vi "MotorBlockPI_FPGA.vi"(1 "Encoder":T1(ring), 3 "STOP":bool, 5 "Value":dbl, 7 "Custom FPGA Reference In":refnum<k20>, 9 "Speed":dbl, 11 "error in (no error)":errorcluster, 12 "Type":enum16{"Iterations", "Counts", "Time"}(ring), 13 "Motor":T2(ring), 14 "Sentido":bool) -> (4 "Waveform \nChart":dbl[][](graph), 10 "FPGA VI Reference Out":refnum<k20>, 15 "error out":errorcluster)   [LabVIEW 2017]
doc: "This program is an PI counts based program usgin only the FPGA customized encoders. \nIt works using counts, degrees, iterations, time or rotations.\nEach iteration delates 5 ms. You must to use with VI without a while loop."
uses:
  <vilib>/Platform/TimedLoop/XDataNode/timing_clust.ctl
  <vilib>/Platform/TimedLoop/XDataNode/nitl_modes.ctl
  <vilib>/Platform/TimedLoop/XDataNode/wakeup.ctl
  <vilib>/Utility/error.llb/Error Cluster From Error Code.vi
  <vilib>/rvi/errors/niLvFpgaAdjustHostInterfaceError.vi
  <vilib>/myRIO/Common/Instrument Driver Framework/myRIO v1.0/DIO/vis/myRIO v1.0 Write DIO.vi
  <vilib>/myRIO/Common/Instrument Driver Framework/myRIO v1.0/PWM/vis/myRIO v1.0 Write PWM.vi
  <vilib>/Platform/TimedLoop/XDataNode/XDataNode.xnode
  <vilib>/rvi/interface/nirviReadWriteControl/nirviReadWriteControl.xnode
  <vilib>/myRIO/Instrument Drivers/Onboard IO/PWM/PWM.lvlib
  <vilib>/myRIO/Instrument Drivers/Onboard IO/DIO/DIO.lvlib
  <vilib>/Platform/TimedLoop/XDataNode/XDNodeRunTimeDep.lvlib
  NiFpgaLv.dll
  <vilib>/rvi/interface/Simulation/niFpgaSimulationCallBeginRW.vi
panel:
  # "Este programa implementa un control por odometría usando únicamente los \nencoders de la FPGA. \nWRO 2018 @ Tecnológico de Costa Rica"
  # "El programa puede hacer funcionar los motores por tiempo, \niteraciones, grados, rotaciones o cuentas puras. \nParametros de entrada:\nType: Selecciona el modo desea para operar el programa:\n        \n            2. Time:     Detiene el motor depués de transcurrido el \n                                tiempo deseado.\n            3. Iteration:     Detiene el motor depués de transcurrido una\n                                cantidad de iteraciones.\n             5. Counts:  Detiene el motor depués de alcanzada la posición \n                                 en cuentas deseada.\nValue: Indica el valor de la condición de parada deseada.\nMotor: Selecciona el puerto y el motor.\nSentido: Selecciona el sentido de giro.\nFPGA Reference In: Selecciona la referencia al programa de FPGA.\nFPGA Reference Out: Envía la referencia al programa de FPGA.\nError I/O: Maneja las entadas y salidas de error.\nEncoder: Selecciona la entrada a utilizar como encoder. Los números \nrepresentan el número de DIO que se deben conectar, y siempre el número \nmás pequeño representa la fase A."
  # "Horario"
  # "Antihorario"
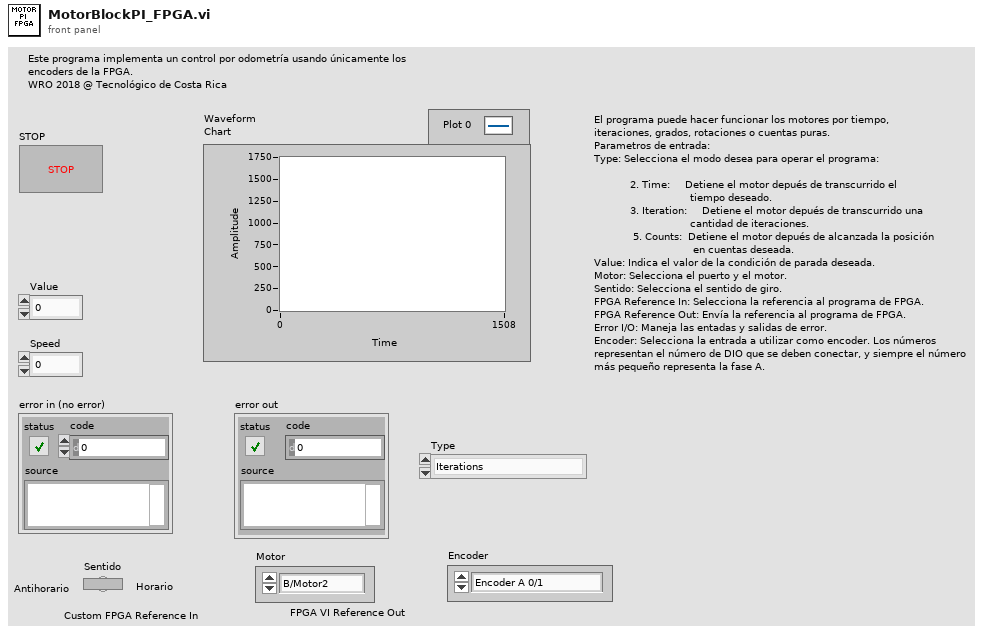
[diagram p1: front panel]
types:
  T1 = enum16{"Encoder A 0/1", "Encoder A 11/12", "Encoder A 4/13", "Encoder B 0/1", "Encoder B 11/12", "Encoder B 4/13", "Encoder C 4/6", "Encoder C 0/2"}
  T2 = enum16{"B/Motor2", "B/Motor1", "A/Motor2", "A/Motor1"}
  T3 = typedef "XDNodeRunTimeDep.lvlib/timing_clust.ctl" = cluster{"Expected End [f-1]":u64, "Actual End [f-1]":u64, "Finished Late? [f-1]":bool, "Expected End [i-1]":u64, "Actual End [i-1]":u64, "Finished Late? [i-1]":bool, "Expected Start [i]":u64, "Actual Start [i]":u64, "Expected Start [f]":u64, "Actual Start [f]":u64, "Source Name":string, "Structure Name":string, "Period":i64, "Deadline":i64, "Offset":i64, "Start":i64, "Priority":i32, "Timeout":i32, "Mode":T4, "Wakeup Reason":T5, "Error":errorcluster, "Source Type":string, "Secondary Source Type":string, "Global End Time":u64, "Global Start Time":u64, "Frame Duration":u64, "Iteration Duration":u64, "Assigned CPU":i32, "I/O Scan Engine Mode":u32}
  T4 = typedef "XDNodeRunTimeDep.lvlib/nitl_modes.ctl" = enum32{"No Change", "Process missed periods, maintain original phase", "Discard missed periods, maintain original phase", "Process missed periods, ignore original phase", "Discard missed periods, ignore original phase"}
  T5 = typedef "XDNodeRunTimeDep.lvlib/wakeup.ctl" = enum32{"Normal", "Aborted", "Asynchronous wakeup", "Timing source error", "Timed loop error", "Timeout"}
  T6 = typedef "DIO.lvlib/DIO Reference.ctl" = cluster{"myRIO Reference":T7, "DIO Channels List":T11}
  T7 = typedef "myRIO Generic Hardware Reference.ctl" = cluster{"myRIO Model":T8, "myRIO Hardware Reference":T9}
  T8 = typedef "Hardware Version Enum.ctl" = enum16{"Unknown", "myRIO-1900", "myRIO-1950", "roboRIO", "NI ELVIS RIO CM"}
  T9 = typedef "myRIO v1.0 Reference.ctl" = cluster{"Generic FPGA Reference":T10, "Allow multiple opens":bool}
  T10 = typedef "Generic FPGA Reference.ctl" = refnum<k20>
  T11 = typedef "DIO Channels List.ctl" = T12[]
  T12 = typedef "DIO Channels Enum.ctl" = enum16{"Not Connected", "C/DIO0", "C/DIO1", "C/DIO2", "C/DIO3", "C/DIO4", "C/DIO5", "C/DIO6", "C/DIO7", "A/DIO0", "A/DIO1", "A/DIO2", "A/DIO3", "A/DIO4", "A/DIO5", "A/DIO6", "A/DIO7", "A/DIO8", "A/DIO9", "A/DIO10", "A/DIO11", "A/DIO12", "A/DIO13", "A/DIO14", "A/DIO15", "B/DIO0", "B/DIO1", "B/DIO2", "B/DIO3", "B/DIO4", "B/DIO5", "B/DIO6", "B/DIO7", "B/DIO8", "B/DIO9", "B/DIO10", "B/DIO11", "B/DIO12", "B/DIO13", "B/DIO14", "B/DIO15", "LED0", "LED1", "LED2", "LED3", "Button0", "DIO/DIO0", "DIO/DIO1", "DIO/DIO2", "DIO/DIO3", "DIO/DIO4", "DIO/DIO5", "DIO/DIO6", "DIO/DIO7", "DIO/DIO8", "DIO/DIO9", "SPI/CS0", "SPI/CS1", "SPI/CS2", "SPI/CS3", "LED RADIO (Green)", "LED RADIO (Red)", "LED COMM (Green)", "LED COMM (Red)", "LED MODE (Green)", "LED MODE (Red)"}
  T13 = typedef "PWM.lvlib/PWM Reference.ctl" = cluster{"myRIO Reference":T7, "PWM Channels Enum":T14, "PWM Configuration":T15}
  T14 = typedef "PWM Channels Enum.ctl" = enum16{"Not Connected", "C/PWM0", "C/PWM1", "A/PWM0", "A/PWM1", "A/PWM2", "B/PWM0", "B/PWM1", "B/PWM2", "PWM/PWM0", "PWM/PWM1", "PWM/PWM2", "PWM/PWM3", "PWM/PWM4", "PWM/PWM5", "PWM/PWM6", "PWM/PWM7", "PWM/PWM8", "PWM/PWM9"}
  T15 = typedef "PWM.lvlib/PWM Configuration.ctl" = cluster{"Frequency":dbl, "Duty Cycle":dbl}
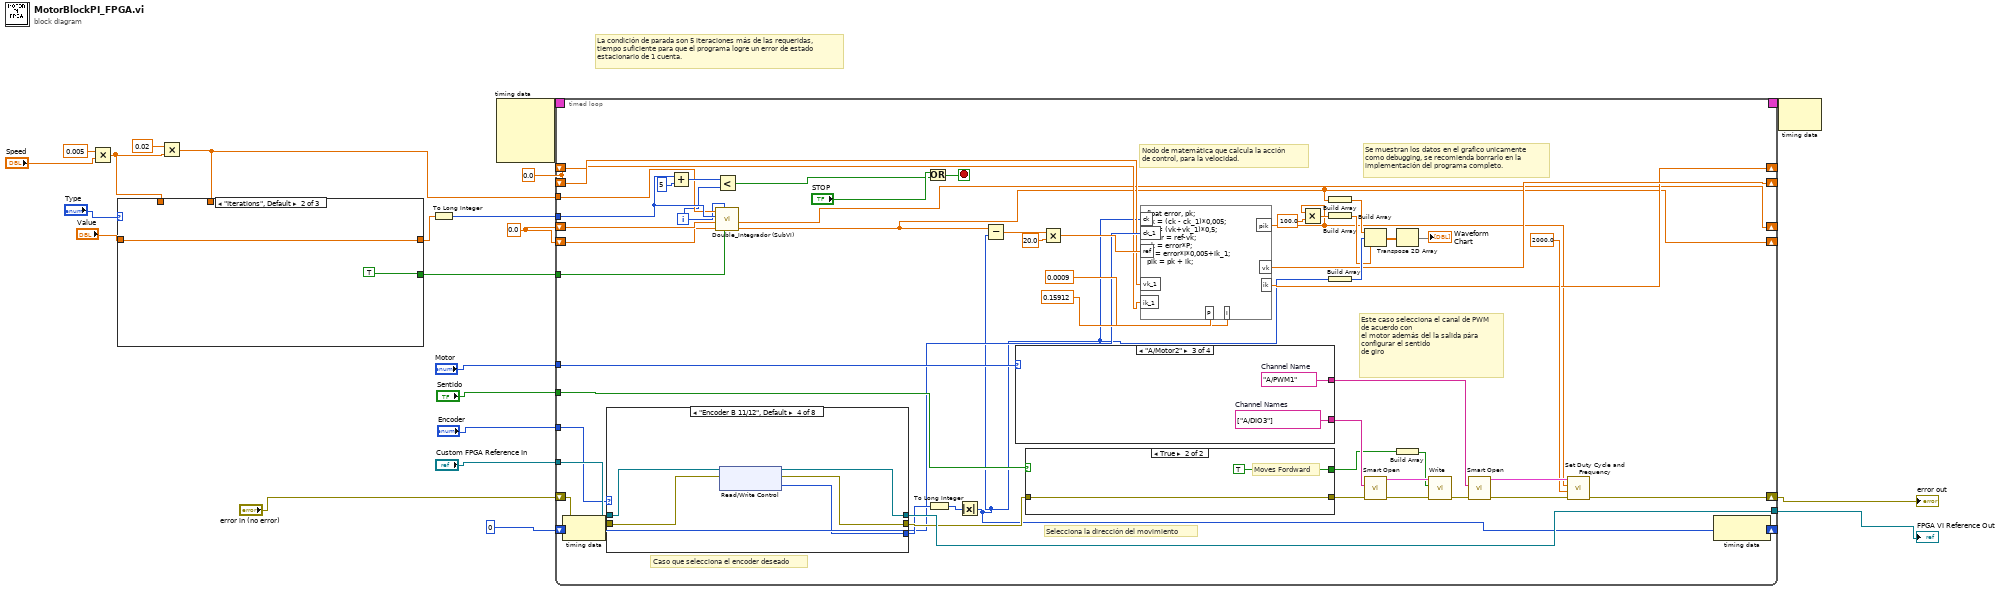
[diagram p0: block diagram]
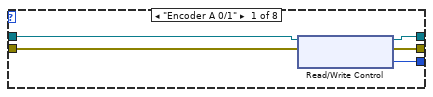
[diagram p2: hidden frame]
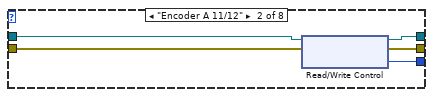
[diagram p3: hidden frame]
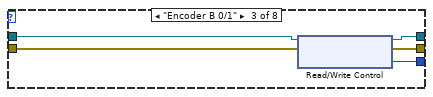
[diagram p4: hidden frame]
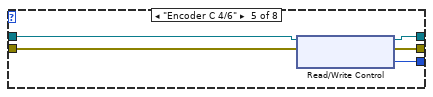
[diagram p5: hidden frame]
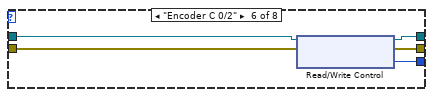
[diagram p6: hidden frame]
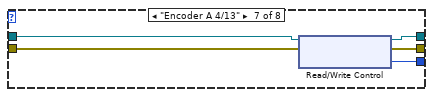
[diagram p7: hidden frame]
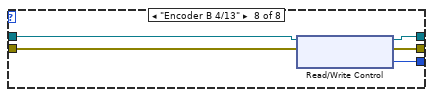
[diagram p8: hidden frame]
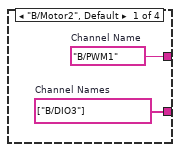
[diagram p9: hidden frame]
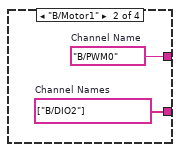
[diagram p10: hidden frame]
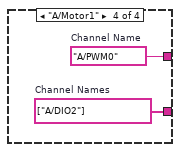
[diagram p11: hidden frame]
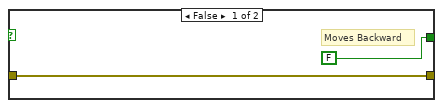
[diagram p12: hidden frame]
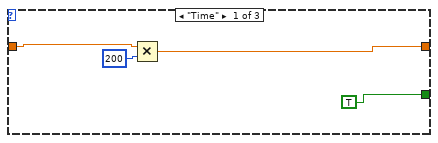
[diagram p13: hidden frame]
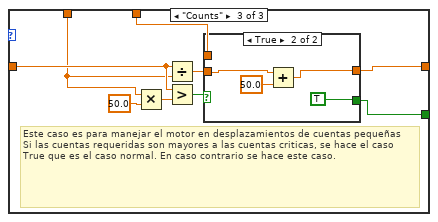
[diagram p14: hidden frame]
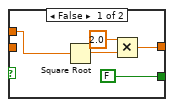
[diagram p15: hidden frame]
diagram:
  w17 = 0.0
  w11 = 0.0
  # "La condición de parada son 5 iteraciones más de las requeridas,\ntiempo suficiente para que el programa logre un error de estado\nestacionario de 1 cuenta."
  n1 = Multiply(x=0.005, y="Speed") -> (x*y=w4:dbl)
  n2 = Multiply(x=0.02, y=w4) -> (x*y=w2:dbl)
  n3 = case shown="\"Iterations\", Default" "Type" {
    tunnel: "Value" -> [w24 w27 w32]
    tunnel: w4 -> [_ _ w30]
    tunnel: [w25 w27 w35] -> w10
    tunnel: [TRUE TRUE w33] -> w8
    tunnel: w2 -> [_ _ w29]
    frame "Time" {
      n4 = Multiply(x=w24, y=200) -> (x*y=w25:dbl)
    }
    frame "Iterations", Default {
    }
    frame "Counts" {
      # "Este caso es para manejar el motor en desplazamientos de cuentas pequeñas\nSi las cuentas requeridas son mayores a las cuentas criticas, se hace el caso True que es el caso normal. En caso contrario se hace este caso."
      n5 = Multiply(x=w30, y=50.0) -> (x*y=w31:dbl)
      n6 = Divide(x=w32, y=w30) -> (x/y=w34:dbl)
      n7 = Greater?(x=w32, y=w31) -> (0:w36:bool)
      n8 = case shown="True" w36 {
        tunnel: [w40 w44] -> w35
        tunnel: w34 -> [_ w43]
        tunnel: [FALSE TRUE] -> w33
        tunnel: w29 -> [w38 _]
        frame False {
          n9 = Square Root(x=w38) -> (sqrt(x)=w42:dbl)
          n10 = Multiply(x=2.0, y=w42) -> (x*y=w40:dbl)
        }
        frame True {
          n11 = Add(x=w43, y=50.0) -> (x+y=w44:dbl)
        }
      }
    }
  }
  n12 = To Long Integer(number=w10) -> (32bit integer=w9:i32)
  n13 = node-c288() -> (w19:T3)  [unwired: 4 in]
  n14 = timed-loop {
    shift-right: [w61] -> _
    shift-left: w11 -> [w60]
    tunnel: w2 -> [w66]
    shift-right: [w91] -> w14
    shift-left: "error in (no error)" -> [w74]
    tunnel: w9 -> [w67]
    tunnel: "Sentido" -> [w99]
    tunnel: "Motor" -> [w83]
    timing: w19 -> [_]
    timing-out: [_] -> w18
    shift-right: [w50] -> _
    shift-left: w17 -> [w65]
    shift-right: [w49] -> _
    shift-left: w17 -> [w64]
    tunnel: "Custom FPGA Reference In" -> [w75]
    tunnel: [w73] -> w15
    tunnel: "Encoder" -> [w56]
    shift-right: [w48] -> _
    shift-left: 0 -> [w63]
    shift-right: [w58] -> _
    shift-left: w11 -> [w59]
    tunnel: w8 -> [w57]
    i -> [w62]
    stop <- w96 stop-if-true
    # "Nodo de matemática que calcula la acción \nde control, para la velocidad."
    # "Se muestran los datos en el grafico unicamente \ncomo debugging, se recomienda borrarlo en la \nimplementación del programa completo."
    # "Este caso selecciona el canal de PWM de acuerdo con \nel motor además del la salida pára configurar el sentido\nde giro"
    # "Selecciona la dirección del movimiento"
    # "Caso que selecciona el encoder deseado"
    n15 = node-c288() -> ()  [unwired: 1 in, 1 out]
    n16 = case shown="\"Encoder B 11/12\", Default" w56 {
      tunnel: w75 -> [w102 w105 w111 w119 w121 w126 w132 w136]
      tunnel: w74 -> [w101 w106 w110 w115 w120 w125 w131 w135]
      tunnel: [w104 w109 w112 w118 w124 w129 w133 w137] -> w73
      tunnel: [w103 w108 w113 w116 w123 w128 w134 w138] -> w72
      tunnel: [w100 w107 w114 w117 w122 w127 w130 w139] -> w70
      frame "Encoder A 0/1" {
        n17 = xnode "Read/Write Control"("FPGA VI Reference In"=w102, "error in"=w101) -> ("FPGA VI Reference Out"=w104:refnum<k20>, "error out"=w103:errorcluster, "ENC.A.CNTR.2"=w100:u32)
      }
      frame "Encoder A 11/12" {
        n18 = xnode "Read/Write Control"("FPGA VI Reference In"=w105, "error in"=w106) -> ("FPGA VI Reference Out"=w109:refnum<k20>, "error out"=w108:errorcluster, "ENC.A.CNTR"=w107:u32)
      }
      frame "Encoder B 0/1" {
        n19 = xnode "Read/Write Control"("FPGA VI Reference In"=w111, "error in"=w110) -> ("FPGA VI Reference Out"=w112:refnum<k20>, "error out"=w113:errorcluster, "ENC.B.CNTR 2"=w114:u32)
      }
      frame "Encoder B 11/12", Default {
        n20 = xnode "Read/Write Control"("FPGA VI Reference In"=w119, "error in"=w115) -> ("FPGA VI Reference Out"=w118:refnum<k20>, "error out"=w116:errorcluster, "ENC.B.CNTR"=w117:u32)
      }
      frame "Encoder C 4/6" {
        n21 = xnode "Read/Write Control"("FPGA VI Reference In"=w121, "error in"=w120) -> ("FPGA VI Reference Out"=w124:refnum<k20>, "error out"=w123:errorcluster, "ENC.C_1.CNTR"=w122:u32)
      }
      frame "Encoder C 0/2" {
        n22 = xnode "Read/Write Control"("FPGA VI Reference In"=w126, "error in"=w125) -> ("FPGA VI Reference Out"=w129:refnum<k20>, "error out"=w128:errorcluster, "ENC.C_0.CNTR"=w127:u32)
      }
      frame "Encoder A 4/13" {
        n23 = xnode "Read/Write Control"("FPGA VI Reference In"=w132, "error in"=w131) -> ("FPGA VI Reference Out"=w133:refnum<k20>, "error out"=w134:errorcluster, "ENCA.CNTR.3"=w130:u32)
      }
      frame "Encoder B 4/13" {
        n24 = xnode "Read/Write Control"("FPGA VI Reference In"=w136, "error in"=w135) -> ("FPGA VI Reference Out"=w137:refnum<k20>, "error out"=w138:errorcluster, "ENC.B.CNTR_4"=w139:u32)
      }
    }
    n25 = Add(x=w67, y=5) -> (x+y=w68:i32)
    n26 = call "Double_Integrador (SubVI).vi"("Mode"=w57, "Iteration"=w62, "Int_2_k_1"=w64, "Int_1_k_1"=w65, "Value"=w67, "Speed"=w66) -> ("Integral 2"=w49:dbl, "Integral 1"=w50:dbl)  [unwired: 4 in]
    n27 = Less?(x=w68, y=w62) -> (x < y?=w97:bool)
    n28 = Or(x="STOP", y=w97) -> (x .or. y?=w96:bool)
    n29 = To Long Integer(number=w70) -> (32bit integer=w71:i32)
    n30 = Absolute Value(x=w71) -> (abs(x)=w48:i32)
    n31 = Subtract(x=w49, y=w48) -> (x-y=w79:dbl)
    n32 = case shown="\"A/Motor2\"" w83 {
      tunnel: [w142 w145 w146 w149] -> w93
      tunnel: [w143 w144 w147 w148] -> w87
      frame "B/Motor2", Default {
        w143 = tag[] ["B/DIO3"]  # Channel Names
        w142 = tag "B/PWM1"  # Channel Name
      }
      frame "B/Motor1" {
        w144 = tag[] ["B/DIO2"]  # Channel Names
        w145 = tag "B/PWM0"  # Channel Name
      }
      frame "A/Motor2" {
        w147 = tag[] ["A/DIO3"]  # Channel Names
        w146 = tag "A/PWM1"  # Channel Name
      }
      frame "A/Motor1" {
        w148 = tag[] ["A/DIO2"]  # Channel Names
        w149 = tag "A/PWM0"  # Channel Name
      }
    }
    n33 = case shown="True" w99 {
      tunnel: w72 -> [w150 w152]
      tunnel: [FALSE ("A/DIO3 (Pin 17)") TRUE ("A/DIO3 (Pin 17)")] -> w86
      tunnel: [w150 w152] -> w85
      frame False {
        # "Moves Backward"
      }
      frame True {
        # "Moves Fordward"
      }
    }
    n34 = Multiply(x=w79, y=20.0) -> (x*y=w78:dbl)
    n35 = formula code="float error, pk;\nvk = (ck - ck_1)*0,005;\nvk = (vk+vk_1)*0,5;\nerror = ref-vk;\npk = error*P;\nik = error*I*0,005+ik_1;\npik = pk + ik;"("ck"=w48, "ck_1"=w63, "vk_1"=w60, "ref"=w78, "I"=0.15912 ("input variable"), "P"=0.0009 ("input variable"), "ik_1"=w59) -> ("vk"=w61:dbl, "ik"=w58:dbl, "pik"=w47:dbl)
    n36 = Multiply(x=w47, y=100.0) -> (x*y=w51:dbl)
    n37 = Build Array(w49) -> (w54:dbl[])
    n38 = Build Array(w51) -> (w53:dbl[])
    n39 = Build Array(w48) -> (w77:i32[])
    n40 = Build Array(w54, w77, w53) -> (w55:dbl[][])
    n41 = call <vilib>:"Smart Open.vi"("error in (no error)"=w85, "Channel Names"=w87) -> ("error out"=w90:errorcluster, "DIO Ref Out"=w89:T6)  [unwired: 8 in]
    n42 = Transpose 2D Array(2D array=w55) -> (transposed array=→"Waveform \nChart":dbl[][])
    n43 = Build Array(w86) -> (w88:bool[])
    n44 = call <vilib>:"Write.vi"("error in (no error)"=w90, "Values"=w88, "DIO Ref In"=w89) -> ("error out"=w84:errorcluster)  [unwired: 6 in, 1 out]
    n45 = call <vilib>:"Smart Open.vi"("error in (no error)"=w84, "Channel Name"=w93) -> ("error out"=w94:errorcluster, "PWM Ref Out"=w95:T13)  [unwired: 8 in]
    n46 = call <vilib>:"Set Duty Cycle and Frequency.vi"("error in (no error)"=w94, "Frequency [Hz]"=2000.0 ("Duty Cycle"), "Duty Cycle"=w47, "PWM Ref In"=w95) -> ("error out"=w91:errorcluster)  [unwired: 5 in, 1 out]
    n47 = node-c288() -> ()  [unwired: 1 in, 1 out]
  }
  "error out" <- w14
  "FPGA VI Reference Out" <- w15
  n48 = node-c288(w18) -> ()  [unwired: 1 out]
